vi "AlliGator Get Sum Image Threshold.vi"(8 "error in (no error)":errorcluster, 9 "Pixel Counts Constraints":T1 {"High Count Pixels Rejection Options"."High Percentile" min=0.0 max=100.0; "Low Count Pixels Rejection Options"."Low Percentile" min=0.0 max=100.0}, 11 "Image in":T4) -> (0 "error out":errorcluster, 1 "Pixel Threshold Low":sgl, 2 "Pixel Threshold High":sgl, 3 "Image out (dup)":T4, 4 "elapsed (relative) seconds":dbl, 5 "Y Resolution":i32, 7 "X Resolution":i32)   [LabVIEW 2021, in "AlliGator Source Image.lvlib"]
doc: "Computes intensity threshold based on the multi-parameter Pixel Rejection criteria."
uses:
  AlliGator Source Image.lvlib
  <vilib>/vision/Image Controls.llb/IMAQ Image.ctl
  Settings/AlliGator Pixel Counts Constraints.ctl
  Settings/AlliGator High Count Pixels Rejection Options.ctl
  Settings/AlliGator Low Count Pixels Rejection Options.ctl
  Time/Time.lvlib
  Image/Image.lvlib
  Settings/AlliGator Settings.lvlib
panel:
  # "see the AlliGator License on the block diagram (Ctrl+E or Window:Show Block Diagram)"
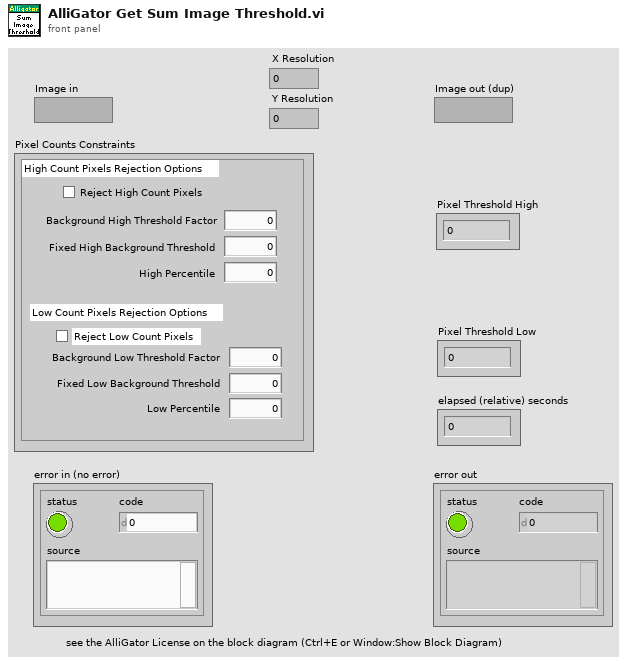
[diagram p1: front panel]
types:
  T1 = typedef "AlliGator Settings.lvlib/AlliGator Pixel Counts Constraints.ctl" = cluster{"High Count Pixels Rejection Options":T2, "Low Count Pixels Rejection Options":T3}
  T2 = typedef "AlliGator Settings.lvlib/AlliGator High Count Pixels Rejection Options.ctl" = cluster{"Background High Threshold Factor":dbl, "Fixed High Background Threshold":dbl, "Reject High Count Pixels":bool, "High Percentile":dbl}
  T3 = typedef "AlliGator Settings.lvlib/AlliGator Low Count Pixels Rejection Options.ctl" = cluster{"Background Low Threshold Factor":dbl, "Fixed Low Background Threshold":dbl, "Reject Low Count Pixels":bool, "Low Percentile":dbl}
  T4 = typedef "IMAQ Image.ctl" = refnum<image>
  T5 = typedef "Image.lvlib/Image Statistics.ctl" = cluster{"Min Value":dbl, "Max Value":dbl, "Mean Value":dbl, "SDV":dbl, "Mode":dbl}
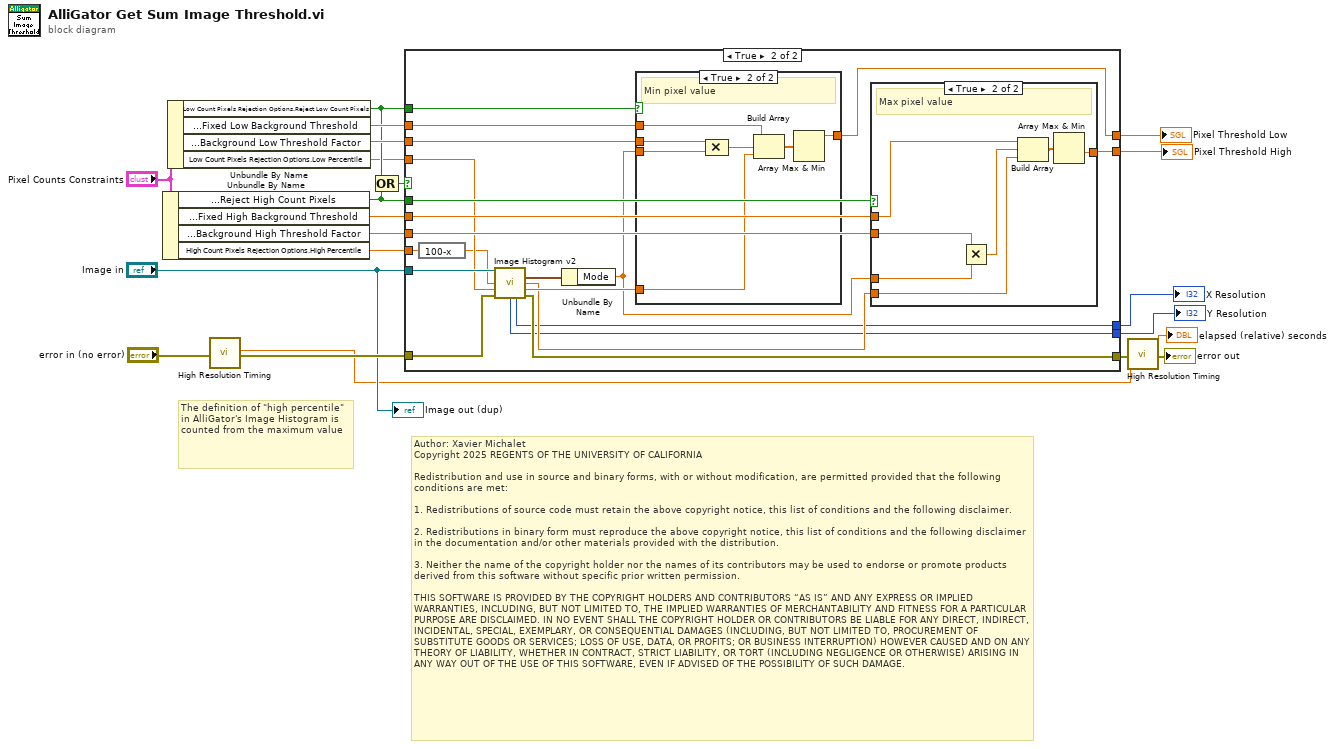
[diagram p0: block diagram]
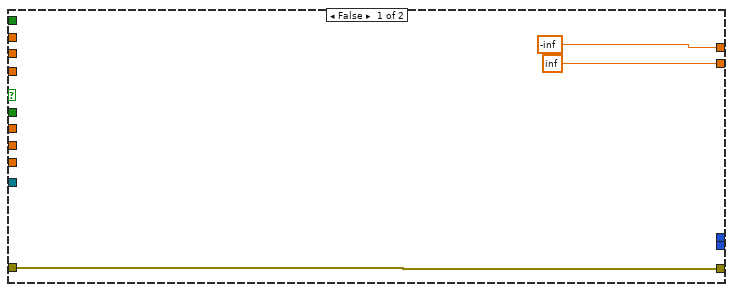
[diagram p2: hidden frame]
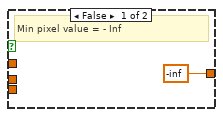
[diagram p3: hidden frame]
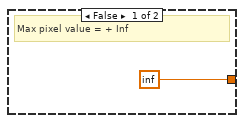
[diagram p4: hidden frame]
diagram:
  # "Author: Xavier Michalet\nCopyright 2025 REGENTS OF THE UNIVERSITY OF CALIFORNIA\n\nRedistribution and use in source and binary forms, with or without modification, are permitted provided that the following conditions are met:\n\n1. Redistributions of source code must retain the above copyright notice, this list of conditions and the following disclaimer.\n\n2. Redistributions in binary form must reproduce the above copyright notice, this list of conditions and the following disclaimer in the documentation and/or other materials provided with the distribution.\n\n3. Neither the name of the copyright holder nor the names of its contributors may be used to endorse or promote products derived from this software without specific prior written permission.\n\nTHIS SOFTWARE IS PROVIDED BY THE COPYRIGHT HOLDERS AND CONTRIBUTORS “AS IS” AND ANY EXPRESS OR IMPLIED WARRANTIES, INCLUDING, BUT NOT LIMITED TO, THE IMPLIED WARRANTIES OF MERCHANTABILITY AND FITNESS FOR A PARTICULAR PURPOSE ARE DISCLAIMED. IN NO EVENT SHALL THE COPYRIGHT HOLDER OR CONTRIBUTORS BE LIABLE FOR ANY DIRECT, INDIRECT, INCIDENTAL, SPECIAL, EXEMPLARY, OR CONSEQUENTIAL DAMAGES (INCLUDING, BUT NOT LIMITED TO, PROCUREMENT OF SUBSTITUTE GOODS OR SERVICES; LOSS OF USE, DATA, OR PROFITS; OR BUSINESS INTERRUPTION) HOWEVER CAUSED AND ON ANY THEORY OF LIABILITY, WHETHER IN CONTRACT, STRICT LIABILITY, OR TORT (INCLUDING NEGLIGENCE OR OTHERWISE) ARISING IN ANY WAY OUT OF THE USE OF THIS SOFTWARE, EVEN IF ADVISED OF THE POSSIBILITY OF SUCH DAMAGE."
  # "The definition of \"high percentile\" in AlliGator's Image Histogram is counted from the maximum value"
  n1 = Unbundle By Name("Pixel Counts Constraints") -> ("High Count Pixels Rejection Options.Reject High Count Pixels"=w9:bool, "High Count Pixels Rejection Options.Fixed High Background Threshold"=w8:dbl, "High Count Pixels Rejection Options.Background High Threshold Factor"=w7:dbl, "High Count Pixels Rejection Options.High Percentile"=w4:dbl)
  n2 = Unbundle By Name("Pixel Counts Constraints") -> ("Low Count Pixels Rejection Options.Reject Low Count Pixels"=w10:bool, "Low Count Pixels Rejection Options.Fixed Low Background Threshold"=w18:dbl, "Low Count Pixels Rejection Options.Background Low Threshold Factor"=w17:dbl, "Low Count Pixels Rejection Options.Low Percentile"=w5:dbl)
  n3 = call "High Resolution Timing.vi"("Error In"="error in (no error)") -> ("elapsed (relative) seconds"=w12:dbl, "Error Out"=w15:errorcluster)  [unwired: 16 in, 1 out]
  n4 = Compound Arithmetic op=OR(w10, w9) -> (w16:bool)
  n5 = case shown="True" w16 {
    tunnel: [-inf w39] -> w21
    tunnel: w18 -> [_ w44]
    tunnel: w17 -> [_ w43]
    tunnel: w15 -> [w24 w42]
    tunnel: [w24 w41] -> w19
    tunnel: "Image in" -> [_ w40]
    tunnel: w10 -> [_ w38]
    tunnel: w9 -> [_ w37]
    tunnel: w8 -> [_ w36]
    tunnel: w7 -> [_ w35]
    tunnel: [inf w34] -> w6
    tunnel: w5 -> [_ w33]
    tunnel: w4 -> [_ w32]
    tunnel: [_ w26] -> w2
    tunnel: [_ w25] -> w1
    frame False {
    }
    frame True {
      n6 = expression code="100-x"(w32) -> (w27:dbl)
      n7 = call "Image Histogram v2.vi"("Image in"=w40, "Max Percentile (0-100)"=w27, "Min Percentile (0-100)"=w33, "Error In"=w42) -> ("Image Statistics"=w29:T5, "Highest Percentile Value"=w30:dbl, "Lowest Percentile Value"=w31:dbl, "Y Resolution"=w25:i32, "X Resolution"=w26:i32, "Error Out"=w41:errorcluster)  [unwired: 5 in, 1 out]
      n8 = Unbundle By Name(w29) -> ("Mode"=w28:dbl)
      n9 = case shown="True" w38 {
        tunnel: w44 -> [_ w52]
        tunnel: w43 -> [_ w50]
        tunnel: [-inf w48] -> w39
        tunnel: w31 -> [_ w47]
        tunnel: w28 -> [_ w46]
        frame False {
          # "Min pixel value = - Inf"
        }
        frame True {
          # "Min pixel value"
          n10 = Compound Arithmetic op=MULTIPLY(w50, w46) -> (w51:dbl)
          n11 = Build Array(w52, w51, w47) -> (w49:dbl[])
          n12 = Array Max & Min(array=w49) -> (max value=w48:dbl)  [unwired: 3 out]
        }
      }
      n13 = case shown="True" w37 {
        tunnel: w36 -> [_ w58]
        tunnel: w35 -> [_ w60]
        tunnel: [inf w56] -> w34
        tunnel: w30 -> [_ w55]
        tunnel: w28 -> [_ w54]
        frame False {
          # "Max pixel value = + Inf"
        }
        frame True {
          # "Max pixel value"
          n14 = Multiply(x=w60, y=w54) -> (x*y=w59:dbl)
          n15 = Build Array(w58, w59, w55) -> (w57:dbl[])
          n16 = Array Max & Min(array=w57) -> (min value=w56:dbl)  [unwired: 3 out]
        }
      }
    }
  }
  "Pixel Threshold Low" <- w21
  "Pixel Threshold High" <- w6
  "X Resolution" <- w2
  "Y Resolution" <- w1
  n17 = call "High Resolution Timing.vi"("relative seconds (NaN)"=w12, "Error In"=w19) -> ("elapsed (relative) seconds"=→"elapsed (relative) seconds":dbl, "Error Out"=→"error out":errorcluster)  [unwired: 15 in, 1 out]
  "Image out (dup)" <- "Image in"
